vi "sv_Build x and y Axes for Octave.vi"(3 "y0 and delta y":cluster{"y0":dbl, "delta y":dbl} {"delta y" format="%.2f"; "y0" format="%.2f"}, 4 "bandedge freq. list":T1(array[cluster]) {"midband" format="%.2f"; "f high" format="%.2f"; "f low" format="%.2f"}, 5 "size(s)":i32[](array[numeric])) -> (0 "y autoscale":cluster{"y min":dbl, "y max":dbl} {"y max" format="%.2f"; "y min" format="%.2f"}, 1 "x autoscale":cluster{"x min":dbl, "x max":dbl} {"x max" format="%.2f"; "x min" format="%.2f"}, 2 "scale info":cluster{"x scale":dbl[], "y scale":dbl[]} {"y scale" format="%.2f"; "x scale" format="%.2f"})   [LabVIEW 2017]
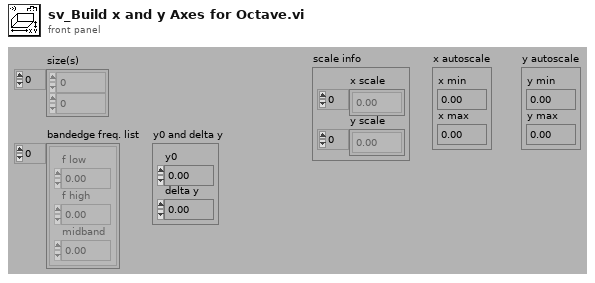
[diagram p1: front panel]
types:
  T1 = cluster{"f low":dbl, "f high":dbl, "midband":dbl}[]
  T2 = cluster{"f low":dbl, "f high":dbl, "midband":dbl}
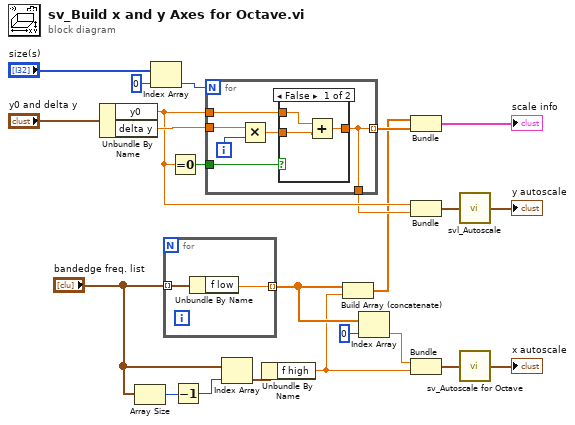
[diagram p0: block diagram]
diagram:
  n1 = Unbundle By Name("y0 and delta y") -> ("y0"=w18:dbl, "delta y"=w23:dbl)
  n2 = Array Size(array="bandedge freq. list") -> (size(s)=w10:i32)
  n3 = Index Array(array="size(s)", index=0) -> (element=w21:i32)
  n4 = for {
    tunnel: "bandedge freq. list" -> [w25] mode=indexing
    tunnel: [w24] -> w3 mode=indexing
    n5 = Unbundle By Name(w25) -> ("f low"=w24:dbl)
  }
  n6 = Equal To 0?(x=w18) -> (x = 0?=w22:bool)
  n7 = Decrement(x=w10) -> (x-1=w6:i32)
  n8 = for {
    N: w21 -> [_]
    tunnel: w22 -> [w31]
    tunnel: w23 -> [w30]
    tunnel: w18 -> [w27]
    tunnel: [w26] -> w15 mode=indexing
    tunnel: [w26] -> w17
    i -> [w29]
    n9 = Multiply(x=w30, y=w29) -> (x*y=w28:dbl)
    n10 = case shown="False" w31 {
      tunnel: w28 -> [w34 w35]
      tunnel: w27 -> [w33 _]
      tunnel: [w32 w35] -> w26
      frame False {
        n11 = Add(x=w33, y=w34) -> (x+y=w32:dbl)
      }
      frame True {
      }
    }
  }
  n12 = Index Array(array="bandedge freq. list", index=w6) -> (element=w8:T2)
  n13 = Unbundle By Name(w8) -> ("f high"=w2:dbl)
  n14 = Build Array (concatenate)(w3, w2) -> (w1:dbl[])
  n15 = Index Array(array=w3, index=0) -> (element=w11:dbl)
  n16 = Bundle(w1, w15) -> (→"scale info":cluster{dbl[], dbl[]})  [unwired: 1 in]
  n17 = Bundle("y0"=w18, w17) -> (w14:cluster{"y0":dbl, dbl})  [unwired: 1 in]
  n18 = Bundle("f low"=w11, "f high"=w2) -> (w5:cluster{"f low":dbl, "f high":dbl})  [unwired: 1 in]
  n19 = call <vilib>:"svl_Autoscale.vi"("scale"=w14) -> ("autoscale"=→"y autoscale":cluster{"min":dbl, "max":dbl})
  n20 = call <vilib>:"sv_Autoscale for Octave.vi"("scale"=w5) -> ("autoscale"=→"x autoscale":cluster{"min":dbl, "max":dbl})
